vi "WildBugChilGru.vi"() -> ()   [LabVIEW 2014]
uses:
  <vilib>/Utility/miscctls.llb/LVPointTypeDef.ctl
  <vilib>/Utility/xml.llb/Write to XML File(string).vi
  <vilib>/Platform/browser.llb/Open URL in Default Browser (string).vi
  <vilib>/Instr/_visa.llb/VISA Configure Serial Port (Instr).vi
  <vilib>/Analysis/3filter.llb/IIR Filter (DBL).vi
  <vilib>/gmath/NI_Gmath.lvlib
  <vilib>/Analysis/NI_AALBase.lvlib
panel:
  in  "Fahrzeugdaten":string
  out "Ergebnis":string
  out "Pmax":string="0,0 PS"
  in  "Drucken":bool
  in  "Speichern":bool
  in  "Start":bool
  in  "Ende":bool
  in  "Spenden":bool
  in  "Registerkarte":T1(tab)
  in  "Zündung [Imp/U]":dbl=1.0
  in  "Übersetzung ermitteln aus":T2(ring)
  in  "Getriebe [1:]":dbl=4.0
  in  "Reifenumfang [m]":dbl=1.2
  in  "Dauer [s]":dbl=5.0
  in  "nKuWe/nRolle":dbl=1.0 format="%#.3f"
  in  "Lufttemperatur [°C]":dbl format="%#.1g"
  in  "Luftdruck [mbar]":dbl=1013.45
  in  "Messung Klimadaten":bool=TRUE
  in  "v vom Gas [km/h]":dbl=5000.0
  in  "Gleitender Mittelwert":u8=35
  in  "Differenzenquotient":u8=12
  in  "n vom Gas [1/min]":dbl=5000.0
  in  "Rollengeber [Inkr/U]":u16=200
  in  "Rollenumfang [m]":dbl=0.613
  in  "Rollenträgheit [kgm²]":dbl=0.402
  in  "Recalc":bool
  in  "Leistung":bool=TRUE caption="Messung Klimadaten"
  out "Datenspeicher":T3={"Fahrzeugdaten"="", "date/time string"="", "Rolle [Inkr/U]"=200, "Rollenumfang [m]"=0.613, "Rollenträgheit [kgm²]"=0.402, "Zündung [Imp/U]"=1.0, "Getriebe [1:]"=4.0, "Reifenumfang [m] "=1.2, "element"=0.0, "Gl. Mittelwert"=35, "Differenzenquotient"=12, 0, "dT [s]"=0.0, "element"=0.0, "Lufttemperatur [°C]"=0.0, "Luftfeuchtigkeit [%]"=43.8, "Luftdruck [mbar]"=1013.45, "nRolle"=[], "nWelle"=[], "ArrayReserve1"=[], "ArrayReserve2"=[], "Übersetzung ermitteln aus"=0, "[s]"=5.0, "nmin [1/min]"=0.0, "nmax [1/min]"=0.0, "n vom Gas [1/min]"=5000.0, "dT-Array [s]"=[], [], "Boolesch"=TRUE, "Serielle Schnittstelle"="COM6", "nKuWe/nRolle"=1.0, "v vom Gas [km/h]"=5000.0}
  out "COM-Fehlerrate":string="0 / 0,0%"
  in  "Konfiguration:":bool
  out "Füllstand Lesepuffer":u64(slide)=1 scale=1.0..100.0
  out "Lesepuffer":string="\n"
  in  "Serielle Schnittstelle":refnum<visa-resource-name>="COM6"
  in  "Registerkarte 2":enum32{"Seite 1", "Seite 2"}(tab)
  out "Text Zündung":string
  out "Text Rolle":string
  in  "Reset Skalierung":bool
  out "Welle\n[1/min]":cluster{dbl, dbl}(knob) scale=0.0..14000.0
  out "Untersetzung\nermittelt":bool
  out "Hinterrad\n[km/h]":dbl(knob) scale=0.0..200.0
  out "XY-Graph":cluster{dbl[], dbl[]}[](graph)
  out "Untersetzung":dbl format="%#.3f"
  out "Untersetzung-Graph":dbl(graph)=198.99999999999997 caption="Untersetzung"
  # "Leistungsmessung:\n1. Drehzahl konstant halten\n2. START [F1]\n3. Drehzahl weiter halten\n4. bei GO: Vollgas\n5. vom Gas gehen"
  # "Untersetzung aus:"
  # "Eingabe <> Messen"
  # "Tacho <> Leistung"
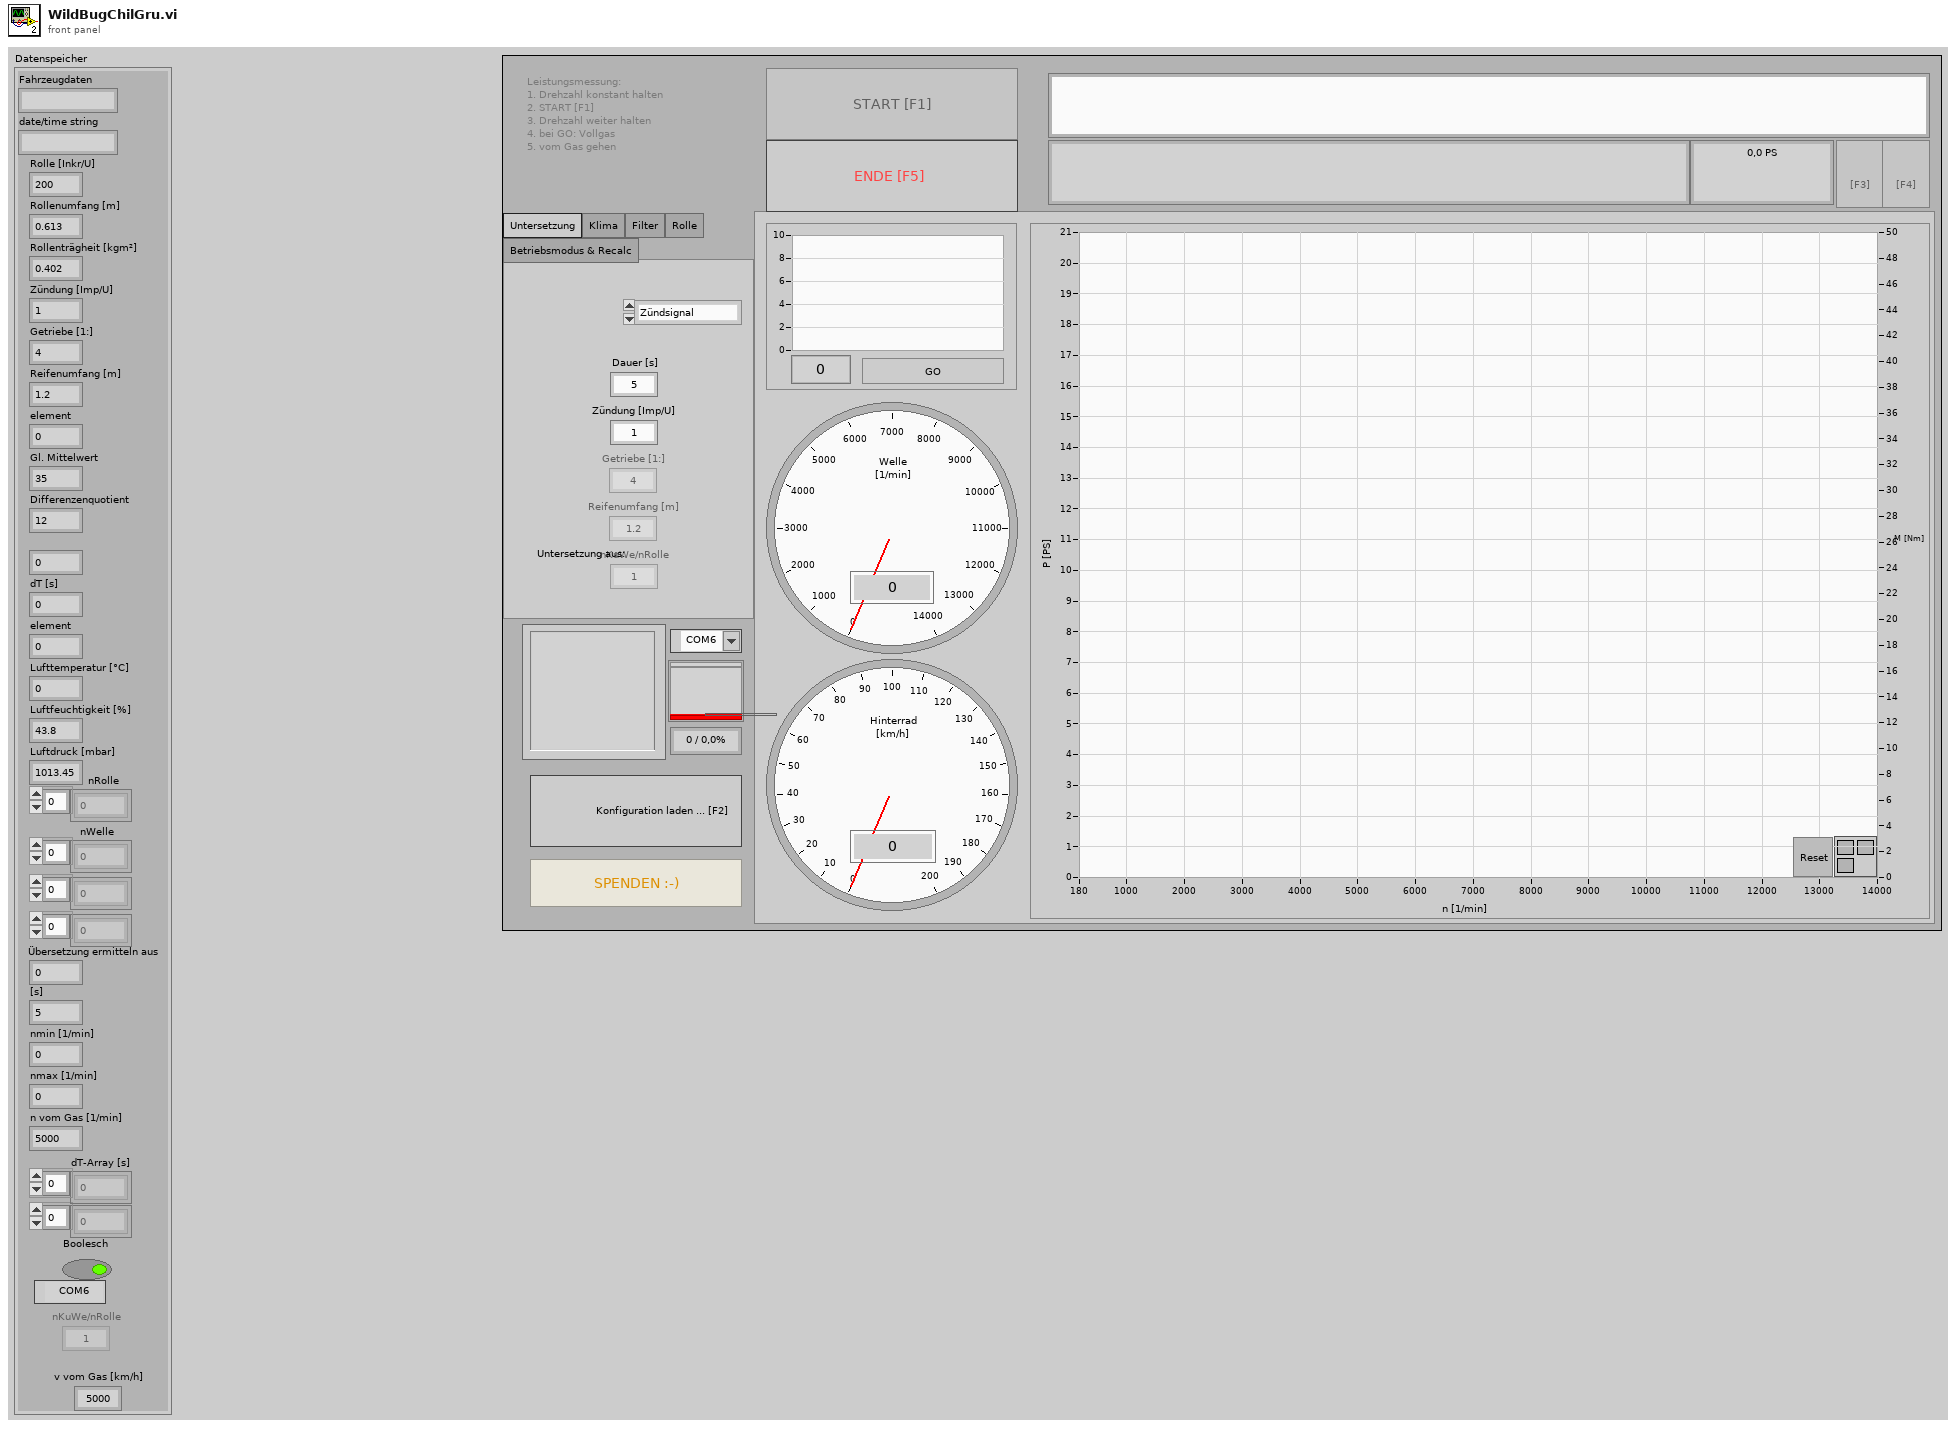
[diagram p1: front panel]
types:
  T1 = enum32{"Untersetzung", "Klima", "Filter", "Rolle", "Betriebsmodus & Recalc"}
  T2 = enum8{"Zündsignal", "Getriebe & Reifen", "nKuWe / nRolle", "Vario (km/h)"}
  T3 = cluster{"Fahrzeugdaten":string, "date/time string":string, "Rolle [Inkr/U]":u16, "Rollenumfang [m]":dbl, "Rollenträgheit [kgm²]":dbl, "Zündung [Imp/U]":dbl, "Getriebe [1:]":dbl, "Reifenumfang [m] ":dbl, "element":dbl, "Gl. Mittelwert":u8, "Differenzenquotient":u8, u8, "dT [s]":dbl, "element":dbl, "Lufttemperatur [°C]":dbl, "Luftfeuchtigkeit [%]":dbl, "Luftdruck [mbar]":dbl, "nRolle":dbl[], "nWelle":dbl[], "ArrayReserve1":dbl[], "ArrayReserve2":dbl[], "Übersetzung ermitteln aus":u8, "[s]":dbl, "nmin [1/min]":dbl, "nmax [1/min]":dbl, "n vom Gas [1/min]":dbl, "dT-Array [s]":dbl[], i32[], "Boolesch":bool, "Serielle Schnittstelle":refnum<visa-resource-name>, "nKuWe/nRolle":dbl, "v vom Gas [km/h]":dbl}
  T4 = enum8{"Enabled", "Disabled", "Disabled and Grayed Out"}
  T5 = cluster{"Fahrzeugdaten":string, "date/time string":string, "Rollengeber [Inkr/U]":u16, "Rollenumfang [m]":dbl, "Rollenträgheit [kgm²]":dbl, "Zündung [Imp/U]":dbl, "Getriebe [1:]":dbl, "Reifenumfang [m] ":dbl, "mean value":dbl, "Gleitender Mittelwert":u8, "Differenzenquotient":u8, u8, dbl, "Numerisch":dbl, "Lufttemperatur [°C]":dbl, dbl, "Luftdruck [mbar]":dbl, dbl[], dbl[], dbl[], dbl[], "Übersetzung ermitteln aus":enum8{"Zündsignal", "Getriebe & Reifen", "nKuWe / nRolle", "Vario (km/h)"}, "Dauer [s]":dbl, dbl, dbl, "n vom Gas [1/min]":dbl, dbl[], i32[], "Messung Klimadaten":bool, "VISA-Referenz (Ausgang)":refnum<visa-resource-name>, "nKuWe/nRolle":dbl, "v vom Gas [km/h]":dbl}
  T6 = typedef "LVPointTypeDef.ctl" = cluster{"Horizontal":i16, "Vertical":i16}
  T7 = enum32{"invalid app kind", "Development System", "Run Time System", "Student Edition", "Embedded LabVIEW", "Evaluation", "Custom"}
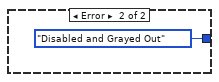
[diagram p8: hidden frame]
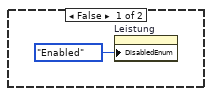
[diagram p9: hidden frame]
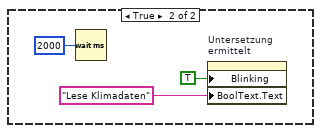
[diagram p10: hidden frame]
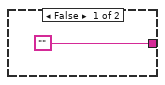
[diagram p12: hidden frame]
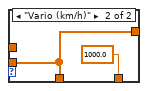
[diagram p15: hidden frame]
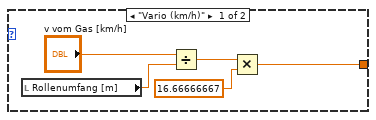
[diagram p16: hidden frame]
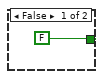
[diagram p17: hidden frame]
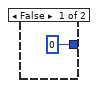
[diagram p19: hidden frame]
diagram:
  n1 = while {
    stop <- w5 stop-if-true
    n2 = local read "Leistung"() -> (w3:bool)
    n3 = Wait (ms)(milliseconds to wait=u32 10) -> ()  [unwired: 1 out]
    n4 = case shown="False" w3 {
      frame False {
        n5 = control-ref of="Welle\n[1/min]"() -> (w9:refnum<vi>)
        n6 = control-ref of="Hinterrad\n[km/h]"() -> (w8:refnum<vi>)
        n7 = control-ref of="Ende"() -> (w7:refnum<vi>)
        n8 = control-ref of="Leistung"() -> (w6:refnum<vi>)
        n9 = call "Tachomodus (SubVI).vi"("Leistung"=w6, "Stopp"=w7, "Hinterrad"=w8, "Welle"=w9) -> ()  [unwired: 8 in]
      }
      frame True {
      }
    }
    n10 = local read "Ende"() -> (w5:bool)
  }
  n11 = while {
    stop <- w13 stop-if-true
    n12 = local read "Start"() -> (w14:bool)
    n13 = Not(x="Leistung") -> (.not. x?=w10:bool)
    n14 = case shown="True" w14 {
      tunnel: "Leistung" -> [_ w23]
      frame False {
        n15 = property on="Leistung" class="Bool. (strikt)"("DisabledEnum"=T4."Enabled" ("Deaktiviert")) -> ()  [unwired: 2 in, 2 out]
      }
      frame True {
        n16 = flat-sequence {
          tunnel: [w115] -> w101
          tunnel: [w114] -> w100
          tunnel: [w112] -> w99
          tunnel: w23 -> [w110]
          tunnel: w101 -> [w129]
          tunnel: w100 -> [w133]
          tunnel: [0] -> w98
          tunnel: [1.0 ("element")] -> w97
          tunnel: [w131] -> w96
          tunnel: [w142] -> w95
          tunnel: [0] -> w94
          tunnel: [w131] -> w93
          tunnel: [-5] -> w92
          tunnel: [w139] -> w91
          tunnel: [w137] -> w90
          tunnel: [w136] -> w89
          tunnel: [0.0] -> w88
          tunnel: [w129] -> w87
          tunnel: [w133] -> w86
          tunnel: w99 -> [w132]
          tunnel: [w132] -> w85
          tunnel: [w170] -> w84
          tunnel: [w169] -> w83
          tunnel: [w168] -> w82
          tunnel: [w167] -> w81
          tunnel: [w166] -> w80
          tunnel: [w165] -> w79
          tunnel: [w164] -> w78
          tunnel: [w163] -> w77
          tunnel: [w162] -> w76
          tunnel: [w161] -> w75
          tunnel: [w160] -> w74
          tunnel: [w159] -> w22
          tunnel: [w158] -> w21
          tunnel: w98 -> [w170]
          tunnel: w97 -> [w169]
          tunnel: w96 -> [w168]
          tunnel: w95 -> [w167]
          tunnel: w94 -> [w166]
          tunnel: w93 -> [w165]
          tunnel: w92 -> [w164]
          tunnel: w91 -> [w163]
          tunnel: w90 -> [w162]
          tunnel: w89 -> [w161]
          tunnel: w88 -> [w160]
          tunnel: w87 -> [w156]
          tunnel: w86 -> [w155]
          tunnel: w85 -> [w157]
          tunnel: w84 -> [w187]
          tunnel: w83 -> [w186]
          tunnel: w82 -> [w185]
          tunnel: w81 -> [w184]
          tunnel: w80 -> [w183]
          tunnel: w79 -> [w182]
          tunnel: w78 -> [w181]
          tunnel: w77 -> [w180]
          tunnel: w76 -> [w179]
          tunnel: w75 -> [w178]
          tunnel: w74 -> [w177]
          tunnel: [w187] -> w73
          tunnel: [w186] -> w72
          tunnel: [w185] -> w71
          tunnel: [w184] -> w70
          tunnel: [w183] -> w69
          tunnel: [w182] -> w68
          tunnel: [w181] -> w67
          tunnel: [w180] -> w66
          tunnel: [w179] -> w65
          tunnel: [w178] -> w64
          tunnel: [w177] -> w63
          tunnel: [w176] -> w62
          tunnel: [w175] -> w61
          tunnel: [w173] -> w60
          tunnel: w22 -> [w176]
          tunnel: w21 -> [w175]
          tunnel: ["Gleitender Mittelwert"] -> w32
          tunnel: [w193] -> w33
          tunnel: [w192] -> w34
          tunnel: [w212] -> w35
          tunnel: [w206] -> w30
          tunnel: [w205] -> w31
          tunnel: [w213] -> w36
          tunnel: [w214] -> w37
          tunnel: [w215] -> w39
          tunnel: [w216] -> _
          tunnel: [w217] -> w41
          tunnel: [w218] -> w42
          tunnel: [w219] -> w55
          tunnel: [w220] -> w18
          tunnel: [w221] -> w57
          tunnel: [w222] -> w58
          tunnel: [w223] -> w59
          tunnel: w73 -> [w223]
          tunnel: w72 -> [w222]
          tunnel: w71 -> [w221]
          tunnel: w70 -> [w220]
          tunnel: w69 -> [w219]
          tunnel: w68 -> [w218]
          tunnel: w67 -> [w217]
          tunnel: w66 -> [w216]
          tunnel: w65 -> [w215]
          tunnel: w64 -> [w214]
          tunnel: w63 -> [w213]
          tunnel: w62 -> [w208]
          tunnel: w61 -> [w207]
          tunnel: w60 -> [w212]
          tunnel: [w199] -> w20
          tunnel: [w200] -> w19
          frame #0 {
            w120 = u16 0 items=["None", "XON/XOFF", "RTS/CTS", "XON/XOFF & RTS/CTS", "DTR/DSR", "XON/XOFF & DTR/DSR"] ("flow control (0:none)")
            w121 = u16 10 items=["1.0"=10, "1.5"=15, "2.0"=20] ("stop bits (10: 1 bit)")
            w113 = FALSE  # Enable Termination Char (T)
            w116 = u32 10000  # timeout (10sec)
            n17 = And(x="Messung Klimadaten", y=w110) -> (x .and. y?=w112:bool)
            n18 = call-poly "VISA Configure Serial Port"("VISA resource name"="Serielle Schnittstelle", "timeout (10sec)"=w116, "Enable Termination\nChar (T)"=w113, "baud rate (9600)"=u32 115200 ("baudrate (250000)"), "data bits (8)"=u16 8, "parity (0:none)"=enum16{"None", "Odd", "Even", "Mark", "Space"}."None", "stop bits (10: 1 bit)"=w121, "flow control (0:none)"=w120) -> ("VISA resource name out"=w118:refnum<visa-resource-name>, "error out"=w117:errorcluster)  [unwired: 6 in]
            n19 = VISA Clear(VISA resource name=w118, error in (no error)=w117) -> (VISA resource name out=w115:refnum<visa-resource-name>, error out=w114:errorcluster)
          }
          frame #1 {
            w130 = T4."Disabled and Grayed Out" ("Deaktiviert")
            w135 = 0.0  # Graphen löschen
            w138 = 0
            w143 = 0.0
            w131 = FALSE
            w136 = ""
            n20 = case shown="False" w132 {
              frame False {
                n21 = property on="Untersetzung\nermittelt" class="Bool. (strikt)"("Blinking"=TRUE ("Blinkend"), "BoolText.Text"="Initialisiere" ("Beschriftung.Text")) -> ()  [unwired: 2 in, 2 out]
              }
              frame True {
                n22 = Wait (ms)(milliseconds to wait=u32 2000 ("Zu wartende ms")) -> ()  [unwired: 1 out]
                n23 = property on="Untersetzung\nermittelt" class="Bool. (strikt)"("Blinking"=TRUE ("Blinkend"), "BoolText.Text"="Lese Klimadaten" ("Beschriftung.Text")) -> ()  [unwired: 2 in, 2 out]
              }
            }
            n24 = Build Array(w135) -> (w125:dbl[])
            n25 = property on="Untersetzung-Graph" class="SVDiagr (strikt)"("History Data"=w125) -> ()  [unwired: 2 in, 2 out]
            n26 = property on="Drucken" class="Bool. (strikt)"("DisabledEnum"=w130) -> ()  [unwired: 2 in, 2 out]
            n27 = property on="Übersetzung ermitteln aus" class="Enum (strikt)"("DisabledEnum"=w130) -> ()  [unwired: 2 in, 2 out]
            n28 = property on="Konfiguration:" class="Bool. (strikt)"("DisabledEnum"=w130) -> ()  [unwired: 2 in, 2 out]
            n29 = property on="Ende" class="Bool. (strikt)"("DisabledEnum"=w130) -> ()  [unwired: 2 in, 2 out]
            n30 = property on="Leistung" class="Bool. (strikt)"("DisabledEnum"=w130) -> ()  [unwired: 2 in, 2 out]
            n31 = property on="Speichern" class="Bool. (strikt)"("DisabledEnum"=w130) -> ()  [unwired: 2 in, 2 out]
            n32 = local write "Pmax"(w136) -> ()
            n33 = local write "COM-Fehlerrate"(w136) -> ()
            n34 = local write "Ergebnis"(w136) -> ()
            n35 = Bundle(w125, w125) -> (w127:cluster{dbl[], dbl[]})  [unwired: 1 in]
            n36 = Bundle(w125, w125) -> (w126:cluster{dbl[], dbl[]})  [unwired: 1 in]
            n37 = Build Array(w127, w126) -> (w128:cluster{dbl[], dbl[]}[])
            n38 = local write "XY-Graph"(w128) -> ()
            n39 = Initialize Array(w138, w138) -> (w137:i32[])
            n40 = Initialize Array(0.0 ("y"), 0) -> (w139:dbl[])
            n41 = Initialize Array(w143, w143) -> (w142:dbl[])
          }
          frame #2 {
            n42 = control-ref of="Lufttemperatur [°C]"() -> (w153:refnum<vi>)
            n43 = control-ref of="Luftdruck [mbar]"() -> (w154:refnum<vi>)
            n44 = call "MessungKlimadaten(SubVI).vi"("Boolesch"=w157, "Fehler (Eingang, kein Fehler)"=w155, "VISA resource name out"=w156, "Lufttemperatur [°C] (Eingang)"=w153, "Luftdruck [mbar] (Eingang)"=w154) -> ("Fehler (Ausgang)"=w158:errorcluster, "VISA-Referenz (Ausgang)"=w159:refnum<visa-resource-name>)  [unwired: 5 in]
          }
          frame #3 {
            n45 = Wait (ms)(milliseconds to wait=u32 2000 ("Zu wartende ms")) -> ()  [unwired: 1 out]
            n46 = call "KorrekturfaktorDin70020 (SubVI).vi"("Lufttemperatur [°C]"="Lufttemperatur [°C]", "Luftdruck [mbar]"="Luftdruck [mbar]") -> ("Numerisch"=w173:dbl)  [unwired: 9 in]
          }
          frame #4 {
            w188 = 0
            n47 = Concatenate Strings("m" ("String"), "\n") -> (w211:string)
            n48 = property on="Untersetzung\nermittelt" class="Bool. (strikt)"("Blinking"=FALSE ("Blinkend")) -> ()  [unwired: 2 in, 2 out]
            n49 = VISA Write(VISA resource name=w208, write buffer=w211, error in (no error)=w207) -> (VISA resource name out=w205:refnum<visa-resource-name>, error out=w206:errorcluster)  [unwired: 1 out]
            n50 = property on="XY-Graph" class="XYGraph (strikt)"("ActYScl"=w188, "YScale.ScaleFit"=w188, "ActYScl"=1, "YScale.ScaleFit"=w188, "XScale.ScaleFit"=w188, "Smooth Update"=TRUE ("Kontinuierliche Aktualisierung")) -> ()  [unwired: 2 in, 2 out]
            n51 = local read "Differenzenquotient"() -> (w203:u8)
            n52 = Divide(x="Gleitender Mittelwert", y=2) -> (x/y=w197:dbl)
            n53 = Round Toward -Infinity(1:w197) -> (0:w198:dbl)
            n54 = call <vilib>:"Smoothing Filter Coefficients.vi"("shape"=1, "half-width"=w198, "type"=0) -> ("forward coefficients"=w193:dbl[], "reverse coefficients"=w192:dbl[])  [unwired: 6 in, 1 out]
            n55 = call <vilib>:"Smoothing Filter Coefficients.vi"("shape"=0, "half-width"=w203, "type"=0) -> ("forward coefficients"=w200:dbl[], "reverse coefficients"=w199:dbl[])  [unwired: 6 in, 1 out]
          }
        }
        n56 = while {
          tunnel: w31 -> [w387]
          tunnel: w30 -> [w386]
          shift-right: [w444] -> _
          shift-left: w37 -> [w400]
          shift-right: [w439] -> _
          shift-left: w36 -> [w443]
          shift-right: [w438] -> _
          shift-left: w36 -> [w442]
          shift-right: [w404] -> _
          shift-left: w36 -> [w441]
          shift-right: [w424] -> _
          shift-left: w59 -> [w440]
          shift-right: [w359] -> w44
          shift-left: w58 -> [_]
          shift-right: [w409] -> w48
          shift-left: w36 -> [w381]
          shift-right: [w377] -> w46
          shift-left: w36 -> [w406]
          shift-right: [w405] -> _
          shift-left: w18 -> [w435]
          shift-right: [w380] -> _
          shift-left: w57 -> [w375]
          shift-right: [w388] -> _
          shift-left: w18 -> [_]
          shift-right: [w365] -> _
          shift-left: w18 -> [_]
          shift-right: [w432] -> w47
          shift-left: w18 -> [w430]
          shift-right: [w431] -> _
          shift-left: w18 -> [w366]
          shift-right: [w371] -> w54
          shift-left: w18 -> [w429]
          shift-right: [w423] -> _
          shift-left: w18 -> [w427]
          shift-right: [w422] -> w24
          shift-left: w18 -> [w428]
          shift-right: [w370] -> w53
          shift-left: w18 -> [w426]
          shift-right: [w369] -> w52
          shift-left: w18 -> [w425]
          tunnel: [w421] -> w56
          shift-right: [w417] -> w51
          shift-left: w55 -> [w419]
          tunnel: [w420] -> w27
          tunnel: [w374] -> w50
          tunnel: ["Rollenumfang [m]"] -> w49
          tunnel: ["Rollenumfang [m]"] -> w43
          shift-right: [w416] -> _
          shift-left: w42 -> [w385]
          shift-right: [w410] -> _
          shift-left: w41 -> [w415]
          shift-right: [w411] -> _
          shift-left: w36 -> [w414]
          shift-right: [w412] -> _
          shift-left: w36 -> [w413]
          shift-right: [w384] -> w40
          shift-left: w18 -> [w408]
          shift-right: [w403] -> _
          shift-left: _ -> [w402]
          shift-right: [w407] -> w38
          shift-left: w39 -> [w401]
          tunnel: [w399] -> w28
          tunnel: w35 -> [w359]
          tunnel: w34 -> [w388]
          tunnel: w33 -> [w365]
          tunnel: w32 -> [w392]
          tunnel: w20 -> [w383]
          tunnel: w19 -> [w382]
          tunnel: [u8 0 ("X-Achse.Achsenanpassung")] -> _
          shift-right: [w357] -> w16
          shift-left: w18 -> [w360]
          i -> [w362]
          stop <- w421 stop-if-true
          n57 = property class="Instr"(reference=w387, error in=w386) -> (reference out=w395:refnum<visa-resource-name>, error out=w394:errorcluster, "Serial Settings:Number of Bytes at Serial Port"=w397:u32)
          n58 = Greater?(x=w397, y=u32 1 ("min. Bytes")) -> (0:w393:bool)
          n59 = case shown="True" w393 {
            tunnel: w397 -> [_ w479]
            tunnel: [u32 0 ("Bytes at Port") w479] -> w396
            frame False {
            }
            frame True {
            }
          }
          n60 = control-ref of="Füllstand Lesepuffer"() -> (w373:refnum<vi>)
          n61 = call "Stringhandling(SubVI)0.0.2.vi"("Slide (Eingang)"=w373, "Numerisch (Eingang)"=w440, "VISA-Referenz (Eingang)"=w395, "MessFrequenz [Hz]"=w441, "Bytes at Port"=w396, "Fehler (Eingang, kein Fehler)"=w394, "Cyclecounter (Eingang)"=w402, "Rolle[Hz]"=w442, "String (Eingang)"=w400, "Zündung [Hz] (Eingang)"=w443) -> ("Lesepuffer"=→"Lesepuffer":string, "Numerisch (Ausgang)"=w424:i32, "String (Ausgang)"=w444:string, "VISA-Referenz (Ausgang)"=w399:refnum<visa-resource-name>, "Zündung [Hz] (Ausgang)"=w439:dbl, "Rolle [Hz]"=w438:dbl, "Messfrequenz [Hz]"=w404:dbl, "Cyclecounter (Ausgang)"=w403:i32, "Fehler (Ausgang)"=w420:errorcluster)  [unwired: 1 in]
          "Füllstand Lesepuffer" <- w424
          n62 = Not Equal?(x=w402, y=w403) -> (x != y?=w389:bool)
          n63 = case shown="True" w389 {
            tunnel: w415 -> [w483 w494]
            tunnel: [w483 w506] -> w410
            tunnel: w414 -> [w482 w505]
            tunnel: [w482 w491] -> w411
            tunnel: w413 -> [w481 w504]
            tunnel: [w481 w492] -> w412
            tunnel: w403 -> [_ w490]
            tunnel: w401 -> [w480 w489]
            tunnel: [w480 w493] -> w407
            frame False {
            }
            frame True {
              n64 = Build Array (concatenate)(w489, w490) -> (w493:i32[])
              n65 = Greater Or Equal To 0?(x=w494) -> (x >= 0?=w495:bool)
              n66 = case shown="True" w495 {
                tunnel: [w507 w518] -> w491
                tunnel: [w507 w519] -> w492
                tunnel: [w508 w510] -> w506
                tunnel: w505 -> [_ w512]
                tunnel: w504 -> [_ w520]
                tunnel: w490 -> [w508 w509]
                tunnel: w494 -> [_ w510]
                frame False {
                  w507 = 1.0
                }
                frame True {
                  w516 = 65536.0
                  n67 = Add(x=w510, y=w512) -> (x+y=w511:dbl)
                  n68 = Divide(x=w511, y=w516) -> (x/y=w521:dbl)
                  n69 = Increment(x=w520) -> (x+1=w519:dbl)
                  n70 = Round Toward -Infinity(1:w521) -> (0:w517:dbl)
                  n71 = Multiply(x=w517, y=w516) -> (x*y=w515:dbl)
                  n72 = Add(x=w515, y=w509) -> (x+y=w514:dbl)
                  n73 = Increment(x=w514) -> (x+1=w513:dbl)
                  n74 = Subtract(x=w513, y=w510) -> (x-y=w518:dbl)
                }
              }
              n75 = Subtract(x=w491, y=w492) -> (x-y=w486:dbl)
              n76 = Decrement(x=w486) -> (x-1=w485:dbl)
              n77 = Max & Min(x=0, y=w485) -> (max(x,y)=w484:dbl)  [unwired: 1 out]
              n78 = Divide(x=w484, y=w491) -> (x/y=w498:dbl)
              n79 = Greater Than 0?(x=w484) -> (x > 0?=w488:bool)
              n80 = Select(t=u32 16711680, s=w488, f=u32 0) -> (s? t:f=w499:u32)
              n81 = Multiply(x=w498, y=100.0) -> (x*y=w496:dbl)
              n82 = property on="COM-Fehlerrate" class="Str"("Text.TextColor"=w499) -> ()  [unwired: 2 in, 2 out]
              n83 = Format Into String(format string="%d / %.1f%%" ("Format-String"), w484, w496) -> (resulting string=→"COM-Fehlerrate":string)  [unwired: 2 in, 1 out]
            }
          }
          n84 = local read "Übersetzung ermitteln aus"() -> (w356:T2)
          n85 = case "Case-Struktur" shown="True" w389 {
            tunnel: w439 -> [w701 w717]
            tunnel: w438 -> [w700 w716]
            tunnel: [w701 w702] -> w437
            tunnel: [w700 w715] -> w436
            tunnel: w404 -> [_ w710]
            tunnel: w381 -> [w699 _]
            tunnel: [w699 w709] -> w409
            tunnel: w406 -> [_ w714]
            tunnel: "Rollenumfang [m]" -> [_ w713]
            tunnel: w356 -> [_ w706]
            frame False {
            }
            frame True {
              w722 = 60.0 ("y")
              n86 = Reciprocal "Abtastzeit [s]"(x=w710) -> (1/x=w709:dbl)
              n87 = Divide "R [1/s]"(x=w716, y="Rollengeber [Inkr/U]") -> (x/y=w721:dbl)
              n88 = Divide(x=w717, y="Zündung [Imp/U]") -> (x/y=w720:dbl)
              n89 = Multiply "nZ gemessen [1/min]"(x=w720, y=w722) -> (x*y=w702:dbl)
              n90 = Multiply "nR [1/min]"(x=w722, y=w721) -> (x*y=w715:dbl)
              n91 = Multiply "nZ berechnet [1/min]"(x=w715, y=w714) -> (x*y=w704:dbl)
              n92 = Multiply "[m/min]"(x=w715, y=w713) -> (x*y=w718:dbl)
              n93 = case shown="Standard" w706 {
                tunnel: [w724 w725] -> w705
                tunnel: w704 -> [w724 w726]
                tunnel: [w723 w726] -> w703
                tunnel: w702 -> [w723 w725]
                frame Default {
                }
                frame "Vario (km/h)" {
                }
              }
              n94 = Multiply "[km/h]"(x=w718, y=0.06) -> (x*y=→"Hinterrad\n[km/h]":dbl)
              n95 = Bundle(w705, w703) -> (→"Welle\n[1/min]":cluster{dbl, dbl})  [unwired: 1 in]
            }
          }
          n96 = case shown="Standard" w356 {
            tunnel: [w470 "n vom Gas [1/min]"] -> w374
            frame "Vario (km/h)" {
              n97 = local read "Rollenumfang [m]"() -> (w471:dbl)
              n98 = Divide(x="v vom Gas [km/h]", y=w471) -> (x/y=w469:dbl)
              n99 = Multiply(x=w469, y=16.66666667) -> (x*y=w470:dbl)
            }
            frame Default {
            }
          }
          n100 = case shown="True" w389 {
            tunnel: w437 -> [_ w551]
            tunnel: w436 -> [_ w616]
            tunnel: "Rollenumfang [m]" -> [_ w619]
            tunnel: [w534 w592] -> w377
            tunnel: w406 -> [w523 w592]
            tunnel: w375 -> [w535 w554]
            tunnel: w435 -> [w536 w622]
            tunnel: [w535 w584] -> w380
            tunnel: [w536 w621] -> w405
            tunnel: w388 -> [_ w618]
            tunnel: w365 -> [_ w617]
            tunnel: [w533 w556] -> w432
            tunnel: [w532 w564] -> w431
            tunnel: w430 -> [w533 w615]
            tunnel: w366 -> [w532 _]
            tunnel: w392 -> [_ w573]
            tunnel: [w531 w597] -> w371
            tunnel: w429 -> [w531 _]
            tunnel: [w530 w563] -> w423
            tunnel: w427 -> [w530 _]
            tunnel: [w529 w598] -> w422
            tunnel: w428 -> [w529 _]
            tunnel: [w528 w609] -> w370
            tunnel: w426 -> [w528 _]
            tunnel: [w527 w608] -> w369
            tunnel: w425 -> [w527 _]
            tunnel: w359 -> [_ w601]
            tunnel: w419 -> [w526 w596]
            tunnel: w374 -> [_ w586]
            tunnel: [w526 w595] -> w417
            tunnel: w385 -> [w525 w591]
            tunnel: [w525 w590] -> w416
            tunnel: w409 -> [_ w589]
            tunnel: [w524 w557] -> w384
            tunnel: w408 -> [w524 w588]
            tunnel: w383 -> [_ w571]
            tunnel: w382 -> [_ w570]
            tunnel: w360 -> [w522 w553]
            tunnel: [w522 w552] -> w357
            frame False {
              n101 = case shown="False" w535 {
                tunnel: w536 -> [w543 _]
                tunnel: [w537 w550] -> w534
                tunnel: w523 -> [_ w550]
                frame False {
                  n102 = call <vilib>:"Measures of Mean.vi"("percent (trim)"=20.0, "type"=3, "x array"=w543) -> ("mean value"=w538:dbl)  [unwired: 7 in, 1 out]
                  n103 = local read "Übersetzung ermitteln aus"() -> (w540:T2)
                  n104 = Equal To 0? "aus Zündsignal?"(x=w540) -> (x = 0?=w539:bool)
                  n105 = case shown="True" w539 {
                    tunnel: w538 -> [w544 w549]
                    tunnel: [w544 w545] -> w537
                    frame False {
                    }
                    frame True {
                      w546 = 1000.0
                      n106 = Multiply(x=w549, y=w546) -> (x*y=w548:dbl)
                      n107 = Round To Nearest(number=w548) -> (nearest integer value=w547:dbl)
                      n108 = Divide(x=w547, y=w546) -> (x/y=w545:dbl)
                    }
                  }
                }
                frame True {
                }
              }
            }
            frame True {
              w604 = 0.00135962  # [W] in [PS]
              w611 = 0.10471975511965978  # 2*Pi/60
              n109 = Not(x=w554) -> (.not. x?=w560:bool)
              n110 = local read "Leistung"() -> (w559:bool)
              n111 = Or(x=w559, y=w560) -> (x .or. y?=w558:bool)
              n112 = Square(x=w592) -> (x^2=w610:dbl)
              n113 = local read "Übersetzung ermitteln aus"() -> (w561:T2)
              n114 = case shown="False" w558 {
                tunnel: w616 -> [_ w634]
                tunnel: w615 -> [w624 w633]
                tunnel: w589 -> [_ w632]
                tunnel: w588 -> [w625 w631]
                tunnel: [w624 w630] -> w556
                tunnel: [w625 w629] -> w557
                tunnel: w553 -> [w623 w628]
                tunnel: [w623 w627] -> w552
                tunnel: w551 -> [_ w626]
                frame False {
                }
                frame True {
                  n115 = Build Array (concatenate) "nRolle in Array einf."(w633, w634) -> (w630:dbl[])
                  n116 = Build Array (concatenate) "dT in Array einf."(w631, w632) -> (w629:dbl[])
                  n117 = Build Array (concatenate) "nWelle in Array einf."(w628, w626) -> (w627:dbl[])
                }
              }
              n118 = Divide(x="Rollenträgheit [kgm²]", y=w610) -> (x/y=w602:dbl)
              n119 = case shown="\"Zündsignal\"" w561 {
                tunnel: w551 -> [w691 _ _ _]
                tunnel: w616 -> [w690 _ _ _]
                tunnel: [w689 w695 "nKuWe/nRolle" 1.0] -> w620
                tunnel: w619 -> [_ w696 _ _]
                frame "Zündsignal" {
                  n120 = Divide(x=w691, y=w690) -> (x/y=w689:dbl)
                }
                frame "Getriebe & Reifen" {
                  n121 = Divide(x=w696, y="Reifenumfang [m]") -> (x/y=w694:dbl)
                  n122 = Multiply(x=w694, y="Getriebe [1:]") -> (x*y=w695:dbl)
                }
                frame "nKuWe / nRolle" {
                }
                frame "Vario (km/h)" {
                }
              }
              n123 = Multiply(x=w602, y=w601) -> (x*y=w600:dbl)
              n124 = local read "Differenzenquotient"() -> (w569:u8)
              n125 = Multiply(x=2, y=w569) -> (x*y=w567:i32)
              n126 = Increment(x=w567) -> (x+1=w565:i32)
              n127 = Index Array(array=w556, index=1 ("Index")) -> (element=w582:dbl)
              n128 = Index Array(array=w557, index=1 ("Index")) -> (element=w576:dbl)
              n129 = Initialize Array(w582, w573) -> (w581:dbl[])
              n130 = Initialize Array(w576, w565) -> (w574:dbl[])
              n131 = Insert Into Array(array=w556, index=0 ("Index"), new element=w581) -> (w579:dbl[])
              n132 = Insert Into Array(array=w557, index=0 ("Index"), new element=w574) -> (w572:dbl[])
              n133 = call-poly <vilib>:"IIR Filter.vi"("Forward Coefficients"=w617, "Reverse Coefficients"=w618, "X"=w579) -> ("Filtered X"=w578:dbl[])  [unwired: 1 in, 1 out]
              n134 = call-poly <vilib>:"IIR Filter.vi"("Forward Coefficients"=w570, "Reverse Coefficients"=w571, "X"=w572) -> ("Filtered X"=w566:dbl[])  [unwired: 1 in, 1 out]
              n135 = case shown="False" w554 {
                selector: w554 -> [_ w688]
                tunnel: w620 -> [w677 _]
                tunnel: w622 -> [w679 w687]
                tunnel: [w674 w688] -> w614
                tunnel: [w678 w687] -> w621
                tunnel: w591 -> [w676 w686]
                tunnel: [w674 w686] -> w590
                tunnel: w561 -> [w673 _]
                frame False {
                  n136 = Build Array (concatenate)(w679, w677) -> (w678:dbl[])
                  n137 = case shown="\"Zündsignal\"" w673 {
                    tunnel: ["Dauer [s]" 0.0 ("Dauer [s]")] -> w675
                    frame "Zündsignal" {
                      n138 = property on="Untersetzung\nermittelt" class="Bool. (strikt)"("Blinking"=TRUE ("Blinkend"), "BoolText.Text"="Ermittle Übersetzung" ("Boolescher Text.Text")) -> ()  [unwired: 2 in, 2 out]
                    }
                    frame Default {
                    }
                  }
                  n139 = call "Verstrichene Zeit"("Time Target (s)"=w675, "Reset"=w676) -> ("Time has Elapsed"=w674:bool)  [unwired: 10 in, 7 out]
                  n140 = case shown="True" w674 {
                    frame False {
                    }
                    frame True {
                      n141 = property on="Untersetzung\nermittelt" class="Bool. (strikt)"("Blinking"=FALSE ("Blinkend"), "BoolText.Text"="Go" ("Boolescher Text.Text")) -> ()  [unwired: 2 in, 2 out]
                    }
                  }
                  "Untersetzung-Graph" <- w677
                }
                frame True {
                }
              }
              n142 = Array Subset "Rolle gefiltert [1/min]"(array=w578, index=w573) -> (w564:dbl[])  [unwired: 1 in]
              n143 = Array Subset "dT gefiltert [s]"(array=w566, index=w565) -> (w562:dbl[])  [unwired: 1 in]
              n144 = Array Size "Array-Größe"(array=w564) -> (size(s)=w612:i32)
              n145 = Greater?(x=w612, y=w573) -> (0:w613:bool)
              n146 = Multiply(x=w564, y=w592) -> (x*y=w597:dbl[])
              n147 = Multiply(x=w597, y=w611) -> (x*y=w563:dbl[])
              n148 = And(x=w614, y=w613) -> (x .and. y?=w584:bool)
              n149 = Array Size "Array-Größe"(array=w563) -> (size(s)=w555:i32)
              n150 = Decrement(x=w555) -> (x-1=w599:i32)
              n151 = Select(t=w586, s=w584, f=1000000.0) -> (s? t:f=w587:dbl)
              n152 = Initialize Array(0.0 ("y"), 0) -> (w605:dbl[])
              n153 = for {
                N: w555 -> [_]
                tunnel: "Differenzenquotient" -> [w649]
                tunnel: w563 -> [w657]
                tunnel: w599 -> [w648]
                shift-right: [w654] -> w598
                shift-left: w605 -> [w655]
                tunnel: w597 -> [w652] mode=indexing
                tunnel: w596 -> [w641]
                tunnel: w587 -> [w651]
                tunnel: [w642] -> w595
                tunnel: w554 -> [w640]
                tunnel: w562 -> [w637] mode=indexing
                i -> [w638]
                stop <- w635 stop-if-true
                n154 = Subtract(x=w648, y=w649) -> (x-y=w650:i32)
                n155 = Multiply(x=w637, y=2.0) -> (x*y=w639:dbl)
                n156 = Subtract(x=w638, y=w649) -> (x-y=w670:i32)
                n157 = Add(x=w638, y=w649) -> (x+y=w664:i32)
                n158 = Greater Or Equal?(x=w638, y=w649) -> (x >= y?=w645:bool)
                n159 = Less Or Equal?(x=w638, y=w650) -> (x <= y?=w646:bool)
                n160 = Greater?(x=w652, y=w651) -> (0:w653:bool)
                n161 = Max & Min(x=w648, y=w664) -> (min(x,y)=w665:i32)  [unwired: 1 out]
                n162 = Max & Min(x=w670, y=0) -> (max(x,y)=w668:i32)  [unwired: 1 out]
                n163 = Subtract(x=w665, y=w638) -> (x-y=w666:i32)
                n164 = Subtract(x=w638, y=w668) -> (x-y=w667:i32)
                n165 = Max & Min(x=w667, y=w666) -> (min(x,y)=w658:i32)  [unwired: 1 out]
                n166 = Add(x=w638, y=w658) -> (x+y=w663:i32)
                n167 = Subtract(x=w638, y=w658) -> (x-y=w662:i32)
                n168 = Multiply(x=w658, y=w639) -> (x*y=w656:dbl)
                n169 = Index Array(array=w657, index=w663) -> (element=w660:dbl)
                n170 = Index Array(array=w657, index=w662) -> (element=w661:dbl)
                n171 = Subtract(x=w660, y=w661) -> (x-y=w659:dbl)
                n172 = Divide(x=w659, y=w656) -> (x/y=w647:dbl)
                n173 = Less Than 0?(x=w647) -> (x < 0?=w644:bool)
                n174 = Less Or Equal To 0?(x=w641) -> (x <= 0?=w643:bool)
                n175 = Build Array (concatenate)(w655, w647) -> (w654:dbl[])
                n176 = Compound Arithmetic op=AND(w644, w653, w643, w645, w646, w640) -> (w635:bool)
                n177 = case shown="False" w635 {
                  tunnel: w638 -> [_ w672]
                  tunnel: [w671 w672] -> w642
                  tunnel: w641 -> [w671 _]
                  frame False {
                  }
                  frame True {
                  }
                }
              }
              n178 = Multiply(x=w598, y=w600) -> (x*y=w609:dbl[])
              n179 = Multiply(x=w563, y=w609) -> (x*y=w603:dbl[])
              n180 = Multiply(x=w604, y=w603) -> (x*y=w608:dbl[])
            }
          }
          "Untersetzung\nermittelt" <- w380
          n181 = local read "Übersetzung ermitteln aus"() -> (w358:T2)
          n182 = Quotient & Remainder(x=w362, y=500) -> (x-y*floor(x/y)=w364:i32)  [unwired: 1 out]
          n183 = Equal To 0? "aus Zündsignal?"(x=w358) -> (x = 0?=w379:bool)
          n184 = Equal To 0?(x=w364) -> (x = 0?=w363:bool)
          n185 = local read "Leistung"() -> (w376:bool)
          n186 = And(x=w380, y=w379) -> (x .and. y?=w378:bool)
          n187 = case shown="True" w376 {
            tunnel: [FALSE w476] -> w418
            tunnel: w417 -> [_ w475]
            frame False {
            }
            frame True {
              n188 = Greater Than 0?(x=w475) -> (x > 0?=w476:bool)
            }
          }
          n189 = case shown="True" w363 {
            tunnel: w371 -> [_ w460]
            tunnel: w370 -> [_ w450]
            tunnel: w369 -> [_ w456]
            tunnel: w358 -> [_ w452]
            tunnel: "Rollenumfang [m]" -> [_ w459]
            tunnel: w357 -> [_ w449]
            frame False {
            }
            frame True {
              # "Skal-Y2"
              # "Skal-Y1"
              # "Skal-X"
              n190 = call "n2v (SubVI).vi"("Übersetzung ermitteln aus"=w452, "Array (Eingang)"=w460, "Rollenumfang [m]"=w459) -> ("Array (Ausgang)"=w453:dbl[])  [unwired: 7 in, 1 out]
              n191 = control-ref of="XY-Graph"() -> (w447:refnum<vi>)
              n192 = case shown="Standard" w452 {
                tunnel: [w465 w467] -> w451
                tunnel: w450 -> [w465 _]
                tunnel: w449 -> [_ w467]
                tunnel: [w465 w467] -> w448
                tunnel: [10.0 1000.0] -> w445
                frame Default {
                }
                frame "Vario (km/h)" {
                }
              }
              n193 = call "Scale_Graph_Y (SubVI).vi"("AktYSkl"=1, "Divisor"=w445, "Array"=w448, "Faktor"=1.8, "XYGraph (Eingang)"=w447) -> ()  [unwired: 7 in]
              n194 = call "Scale_Graph_Y (SubVI).vi"("AktYSkl"=0, "Divisor"=10.0, "Array"=w456, "Faktor"=1.0, "XYGraph (Eingang)"=w447) -> ()  [unwired: 7 in]
              n195 = Bundle("Array (Ausgang)"=w453, w451) -> (w461:cluster{"Array (Ausgang)":dbl[], dbl[]})  [unwired: 1 in]
              n196 = Bundle("Array (Ausgang)"=w453, w456) -> (w462:cluster{"Array (Ausgang)":dbl[], dbl[]})  [unwired: 1 in]
              n197 = call "Scale_Graph_X (SubVI).vi"("Array"=w453, "Übersetzung ermitteln aus"=w452, "XYGraph (Eingang)"=w447) -> ()  [unwired: 9 in]
              n198 = Build Array(w462, w461) -> (w463:cluster{"Array (Ausgang)":dbl[], dbl[]}[])
              n199 = local write "XY-Graph"(w463) -> ()
            }
          }
          n200 = Select(t=w377, s=w380, f=0.0) -> (s? t:f=→"Untersetzung":dbl)
          n201 = case shown="True" w378 {
            tunnel: w377 -> [_ w477]
            frame False {
            }
            frame True {
              n202 = local write "nKuWe/nRolle"(w477) -> ()
            }
          }
          n203 = local read "Start"() -> (w391:bool)
          n204 = Not(x=w391) -> (.not. x?=w390:bool)
          n205 = Or(x=w418, y=w390) -> (x .or. y?=w421:bool)
        }
        n206 = VISA Clear(VISA resource name=w28, error in (no error)=w27) -> (VISA resource name out=w25:refnum<visa-resource-name>, error out=w29:errorcluster)
        n207 = VISA Close(VISA resource name=w25, error in (no error)=w29) -> ()  [unwired: 1 out]
        n208 = case shown="True" w56 {
          tunnel: w54 -> [_ w333]
          tunnel: w53 -> [_ w338]
          tunnel: w52 -> [_ w337]
          tunnel: w51 -> [_ w321]
          tunnel: w24 -> [_ w334]
          tunnel: w50 -> [_ w332]
          tunnel: w49 -> [_ w295]
          tunnel: w44 -> [_ w308]
          tunnel: ["" w305] -> w45
          tunnel: w46 -> [_ w302]
          tunnel: w16 -> [_ w281]
          tunnel: w16 -> [_ w276]
          frame False {
          }
          frame True {
            w293 = 1
            w286 = 0
            w296 = 0.06
            n209 = Array Subset "P"(array=w337, length=w321) -> (w329:dbl[])  [unwired: 1 in]
            n210 = Array Subset "M"(array=w338, length=w321) -> (w330:dbl[])  [unwired: 1 in]
            n211 = Array Subset "alpha"(array=w334, length=w321) -> (w335:dbl[])  [unwired: 1 in]
            n212 = Array Subset "n"(array=w333, length=w321) -> (w331:dbl[])  [unwired: 1 in]
            n213 = property on="Ergebnis" class="Str"("Text.FontSize"=18) -> ()  [unwired: 2 in, 2 out]
            n214 = Array Size(array=w335) -> (size(s)=w336:i32)
            n215 = Array Max & Min "nWellemax [1/min]"(array=w276) -> (max value=w277:dbl)  [unwired: 3 out]
            n216 = for {
              N: w336 -> [w355]
              tunnel: w334 -> [w352]
              tunnel: w333 -> [w349]
              tunnel: w332 -> [w346]
              tunnel: [w344] -> w320
              i -> [w350]
              stop <- w345 stop-if-true
              n217 = Decrement(x=w355) -> (x-1=w354:i32)
              n218 = Subtract(x=w354, y=w350) -> (x-y=w344:i32)
              n219 = Index Array(array=w349, index=w344) -> (element=w348:dbl)
              n220 = Index Array(array=w352, index=w344) -> (element=w353:dbl)
              n221 = Less?(x=w348, y=w346) -> (x < y?=w347:bool)
              n222 = Less Or Equal To 0?(x=w353) -> (x <= 0?=w351:bool)
              n223 = And(x=w351, y=w347) -> (x .and. y?=w345:bool)
            }
            n224 = local read "Übersetzung ermitteln aus"() -> (w284:T2)
            n225 = Increment(x=w320) -> (x+1=w319:i32)
            n226 = Array Subset "M"(array=w330, index=w319) -> (w282:dbl[])  [unwired: 1 in]
            n227 = Array Subset "n"(array=w331, index=w319) -> (w313:dbl[])  [unwired: 1 in]
            n228 = Array Max & Min "Mmax"(array=w282) -> (max value=w280:dbl, max index (indices)=w316:i32)  [unwired: 2 out]
            n229 = Array Max & Min "nmax [1/min]"(array=w313) -> (max value=w278:dbl)  [unwired: 3 out]
            n230 = Array Subset "P"(array=w329, index=w319) -> (w314:dbl[])  [unwired: 1 in]
            n231 = Index Array "n(Mmax)"(array=w313, index=w316) -> (element=w310:dbl)
            n232 = Array Max & Min "Pmax"(array=w314) -> (max value=w311:dbl, max index (indices)=w315:i32)  [unwired: 2 out]
            n233 = case shown="\"Vario (km/h)\"" w284 {
              tunnel: [w341 w343] -> w283
              tunnel: w282 -> [w341 _]
              tunnel: w281 -> [_ w343]
              tunnel: w280 -> [w340 _]
              tunnel: [w340 w342] -> w279
              tunnel: w277 -> [_ w342]
              frame Default {
              }
              frame "Vario (km/h)" {
              }
            }
            n234 = Index Array "n(Pmax)"(array=w313, index=w315) -> (element=w301:dbl)
            n235 = Divide(x=w278, y=w302) -> (x/y=w328:dbl)
            n236 = call "n2v (SubVI).vi"("Übersetzung ermitteln aus"=w284, "Array (Eingang)"=w313, "Rollenumfang [m]"=w295) -> ("Array (Ausgang)"=w312:dbl[], "Boolesch"=w297:bool)  [unwired: 7 in]
            n237 = local read "Lufttemperatur [°C]"() -> (w307:dbl)
            n238 = local read "Luftdruck [mbar]"() -> (w306:dbl)
            n239 = Format Into String(format string="%.1f PS" ("Format-String"), w311) -> (resulting string=→"Pmax":string)  [unwired: 2 in, 1 out]
            n240 = Compound Arithmetic op=MULTIPLY "v(Pmax)"(w301, w295, w296) -> (w303:dbl)
            n241 = Compound Arithmetic op=MULTIPLY "vmax"(w328, w295, w296) -> (w309:dbl)
            n242 = Format Date/Time String(time format string (%c)="%x %H:%M ") -> (date/time string=w305:string)  [unwired: 2 in]
            n243 = Format Into String(format string="%.1f PS bei %d 1/min   |   %.1f Nm bei %d 1/min   |   vmax: %d km/h\\nDIN 70020 k =%.3f (%d \\B0C, %d mbar)\\n%s" ("Format-String"), w311, w301, w280, w310, w309, w308, w307, w306, w305) -> (resulting string=w300:string)  [unwired: 2 in, 1 out]
            n244 = Format Into String(format string="%.1f PS bei %d km/h   |   vmax: %d km/h\\nDIN 70020 k =%.3f (%d \\B0C, %d mbar)\\n%s" ("Format-String"), w311, w303, w309, w308, w307, w306, w305) -> (resulting string=w298:string)  [unwired: 2 in, 1 out]
            n245 = Bundle("Array (Ausgang)"=w312, w314) -> (w318:cluster{"Array (Ausgang)":dbl[], dbl[]})  [unwired: 1 in]
            n246 = Bundle("Array (Ausgang)"=w312, w283) -> (w317:cluster{"Array (Ausgang)":dbl[], dbl[]})  [unwired: 1 in]
            n247 = control-ref of="XY-Graph"() -> (w294:refnum<vi>)
            n248 = Multiply(x=1.8, y=w279) -> (x*y=w292:dbl)
            n249 = Select(t=w298, s=w297, f=w300) -> (s? t:f=→"Ergebnis":string)
            n250 = Build Array(w318, w317) -> (→"XY-Graph":cluster{"Array (Ausgang)":dbl[], dbl[]}[])
            n251 = property on="Eigenschaftsknoten" class="XYGraph (strikt)"(reference=w294, "ActYScl"=w286, "YScale.ScaleFit"=w293, "XScale.ScaleFit"=w293, "ActYScl"=w293, "YScale.Maximum"=w292, "YScale.Minimum"=w286) -> (reference out=w290:refnum<vi>)  [unwired: 1 in, 1 out]
            n252 = property on="Eigenschaftsknoten" class="XYGraph (strikt)"(reference=w290, "ActYScl"=w286) -> (reference out=w287:refnum<vi>, "YScale.Maximum"=w289:dbl)  [unwired: 1 in, 1 out]
            n253 = Add(x=w289, y=3.0) -> (x+y=w285:dbl)
            n254 = property on="Eigenschaftsknoten" class="XYGraph (strikt)"(reference=w287, "ActYScl"=w286, "YScale.Maximum"=w285) -> ()  [unwired: 1 in, 2 out]
            n255 = property on="Pmax" class="Str"("Text.FontSize"=48) -> ()  [unwired: 2 in, 2 out]
          }
        }
        n256 = flat-sequence {
          tunnel: w38 -> [w229]
          tunnel: w40 -> [w230]
          tunnel: w43 -> [w231]
          tunnel: w44 -> [w232]
          tunnel: w45 -> [w233]
          tunnel: w46 -> [w234]
          tunnel: w47 -> [w235]
          tunnel: w48 -> [w236]
          tunnel: [w236] -> w109
          tunnel: [w235] -> w108
          tunnel: [w234] -> w107
          tunnel: [w233] -> w106
          tunnel: [w232] -> w105
          tunnel: [w231] -> w104
          tunnel: [w230] -> w103
          tunnel: [w229] -> w102
          tunnel: [w225] -> w26
          tunnel: w25 -> [w225]
          tunnel: [w224] -> w17
          tunnel: w16 -> [w224]
          tunnel: w109 -> [w266]
          tunnel: w108 -> [w265]
          tunnel: w107 -> [w264]
          tunnel: w106 -> [w263]
          tunnel: w105 -> [w262]
          tunnel: w104 -> [w261]
          tunnel: w103 -> [w260]
          tunnel: w102 -> [w259]
          tunnel: w26 -> [w243]
          tunnel: w17 -> [w237]
          frame #0 {
            w227 = FALSE ("Start [F1]")
            w228 = 0  # Aktivieren
            n257 = local write "Start"(w227) -> ()
            n258 = property on="Drucken" class="Bool. (strikt)"("DisabledEnum"=w228) -> ()  [unwired: 2 in, 2 out]
            n259 = property on="Übersetzung ermitteln aus" class="Enum (strikt)"("DisabledEnum"=w228) -> ()  [unwired: 2 in, 2 out]
            n260 = property on="Speichern" class="Bool. (strikt)"("DisabledEnum"=w228) -> ()  [unwired: 2 in, 2 out]
            n261 = property on="Konfiguration:" class="Bool. (strikt)"("DisabledEnum"=w228) -> ()  [unwired: 2 in, 2 out]
            n262 = property on="Ende" class="Bool. (strikt)"("DisabledEnum"=w228) -> ()  [unwired: 2 in, 2 out]
            n263 = property on="Untersetzung\nermittelt" class="Bool. (strikt)"("BoolText.Text"="GO" ("Boolescher Text.Text"), "Blinking"=w227) -> ()  [unwired: 2 in, 2 out]
            n264 = local write "Untersetzung\nermittelt"(w227) -> ()
          }
          frame #1 {
            w238 = dbl[] []
            w241 = 0.0
            n265 = disable-structure shown="Deaktiviert" {
              frame Disabled {
                n266 = property on="XY-Graph" class="XYGraph (strikt)"("ActYScl"=0, "ActYScl"=1) -> ("XScale.Maximum"=w272:dbl, "XScale.Minimum"=w271:dbl, "YScale.Maximum"=w270:dbl, "YScale.Minimum"=w269:dbl, "YScale.Maximum"=w268:dbl, "YScale.Minimum"=w267:dbl)  [unwired: 2 in, 2 out]
                n267 = Build Array(w272, w271, w270, w269, w268, w267) -> ()  [unwired: 1 out]
              }
              frame Enabled {
              }
            }
            n268 = local read "Gleitender Mittelwert"() -> (w252:u8)
            n269 = local read "Differenzenquotient"() -> (w251:u8)
            n270 = local read "Übersetzung ermitteln aus"() -> (w248:T2)
            n271 = local read "Rollenträgheit [kgm²]"() -> (w256:dbl)
            n272 = local read "Messung Klimadaten"() -> (w245:bool)
            n273 = local read "Rollengeber [Inkr/U]"() -> (w257:u16)
            n274 = local read "Lufttemperatur [°C]"() -> (w250:dbl)
            n275 = local read "Reifenumfang [m]"() -> (w253:dbl)
            n276 = local read "n vom Gas [1/min]"() -> (w246:dbl)
            n277 = local read "Zündung [Imp/U]"() -> (w255:dbl)
            n278 = local read "v vom Gas [km/h]"() -> (w240:dbl)
            n279 = local read "Luftdruck [mbar]"() -> (w249:dbl)
            n280 = local read "nKuWe/nRolle"() -> (w242:dbl)
            n281 = local read "Getriebe [1:]"() -> (w254:dbl)
            n282 = local read "Dauer [s]"() -> (w247:dbl)
            n283 = Bundle("Fahrzeugdaten"="Fahrzeugdaten", "date/time string"=w263, "Rollengeber [Inkr/U]"=w257, "Rollenumfang [m]"=w261, "Rollenträgheit [kgm²]"=w256, "Zündung [Imp/U]"=w255, "Getriebe [1:]"=w254, "Reifenumfang [m]"=w253, "mean value"=w264, "Gleitender Mittelwert"=w252, "Differenzenquotient"=w251, u8 0, w266, "Numerisch"=w262, "Lufttemperatur [°C]"=w250, w241, "Luftdruck [mbar]"=w249, w265, w237, w238, w238, "Übersetzung ermitteln aus"=w248, "Dauer [s]"=w247, w241, w241, "n vom Gas [1/min]"=w246, w260, w259, "Messung Klimadaten"=w245, "VISA-Referenz (Ausgang)"=w243, "nKuWe/nRolle"=w242, "v vom Gas [km/h]"=w240) -> (→"Datenspeicher":T5)  [unwired: 1 in]
          }
        }
      }
    }
    n284 = Boolean To (0,1)(Boolean=w10) -> (0, 1=w12:i16)
    n285 = property on="Registerkarte 2" class="RKElem (strikt)"("Value"=w12) -> ()  [unwired: 2 in, 2 out]
    n286 = local read "Ende"() -> (w13:bool)
  }
  n287 = flat-sequence {
    frame #0 {
      n288 = local read "Datenspeicher"() -> (w727:T3)
      n289 = call <vilib>:"Application Directory.vi"() -> ("Application Directory"=w750:path)
      n290 = Build Path(base path=w750, name or relative path="Konfig.xml") -> (appended path=w729:path)
      n291 = call "LoadCluster(SubVI)2.0.5.vi"("Datenspeicher"=w727, "XML File Path"=w729) -> ("Value"=w728:T3)  [unwired: 8 in, 1 out]
      n292 = property on="Datenspeicher" class="Cluster (strikt)"("Value"=w728) -> ()  [unwired: 2 in, 2 out]
      n293 = Unbundle(w728) -> ("Fahrzeugdaten"=w748:string, "Rolle [Inkr/U]"=w747:u16, "Rollenumfang [m]"=w746:dbl, "Rollenträgheit [kgm²]"=w745:dbl, "Zündung [Imp/U]"=w744:dbl, "Getriebe [1:]"=w743:dbl, "Reifenumfang [m]"=w742:dbl, "element"=w733:dbl, "Gl. Mittelwert"=w741:u8, "Differenzenquotient"=w740:u8, "Lufttemperatur [°C]"=w739:dbl, "Luftdruck [mbar]"=w738:dbl, "Übersetzung ermitteln aus"=w735:u8, "[s]"=w737:dbl, "n vom Gas [1/min]"=w736:dbl, "Boolesch"=w734:bool, "Serielle Schnittstelle"=w732:refnum<visa-resource-name>, "nKuWe/nRolle"=w731:dbl, "v vom Gas [km/h]"=w730:dbl)  [unwired: 13 out]
      n294 = property on="Dauer [s]" class="DigWert (strikt)"("Value"=w737) -> ()  [unwired: 2 in, 2 out]
      n295 = property on="Fahrzeugdaten" class="Str"("Value"=w748) -> ()  [unwired: 2 in, 2 out]
      n296 = property on="Rollengeber [Inkr/U]" class="DigWert (strikt)"("Value"=w747) -> ()  [unwired: 2 in, 2 out]
      n297 = property on="Rollenumfang [m]" class="DigWert (strikt)"("Value"=w746) -> ()  [unwired: 2 in, 2 out]
      n298 = property on="Rollenträgheit [kgm²]" class="DigWert (strikt)"("Value"=w745) -> ()  [unwired: 2 in, 2 out]
      n299 = property on="Zündung [Imp/U]" class="DigWert (strikt)"("Value"=w744) -> ()  [unwired: 2 in, 2 out]
      n300 = property on="Getriebe [1:]" class="DigWert (strikt)"("Value"=w743) -> ()  [unwired: 2 in, 2 out]
      n301 = property on="Reifenumfang [m]" class="DigWert (strikt)"("Value"=w742) -> ()  [unwired: 2 in, 2 out]
      n302 = property on="nKuWe/nRolle" class="DigWert (strikt)"("Value"=w733) -> ()  [unwired: 2 in, 2 out]
      n303 = property on="Gleitender Mittelwert" class="DigWert (strikt)"("Value"=w741) -> ()  [unwired: 2 in, 2 out]
      n304 = property on="Differenzenquotient" class="DigWert (strikt)"("Value"=w740) -> ()  [unwired: 2 in, 2 out]
      n305 = property on="Lufttemperatur [°C]" class="DigWert (strikt)"("Value"=w739) -> ()  [unwired: 2 in, 2 out]
      n306 = property on="Luftdruck [mbar]" class="DigWert (strikt)"("Value"=w738) -> ()  [unwired: 2 in, 2 out]
      n307 = property on="Übersetzung ermitteln aus" class="Enum (strikt)"("Val(Sgnl)"=w735) -> ()  [unwired: 2 in, 2 out]
      n308 = property on="n vom Gas [1/min]" class="DigWert (strikt)"("Value"=w736) -> ()  [unwired: 2 in, 2 out]
      n309 = property on="Messung Klimadaten" class="Bool. (strikt)"("Val(Sgnl)"=w734) -> ()  [unwired: 2 in, 2 out]
      n310 = local write "Serielle Schnittstelle"(w732) -> ()
      n311 = property on="nKuWe/nRolle" class="DigWert (strikt)"("Value"=w731) -> ()  [unwired: 2 in, 2 out]
      n312 = property on="v vom Gas [km/h]" class="DigWert (strikt)"("Value"=w730) -> ()  [unwired: 2 in, 2 out]
      n313 = disable-structure shown="Deaktiviert" {
        disable-tunnel: _ -> [w754 _]
        frame Disabled {
          n314 = Array Size(array=w754) -> (size(s)=w753:i32)
          n315 = Equal?(x=w753, y=6) -> (x = y?=w752:bool)
          n316 = case shown="True" w752 {
            tunnel: w754 -> [_ w755]
            frame False {
            }
            frame True {
              n317 = Index Array(array=w755, index=2) -> (element=w759)
              n318 = Index Array(array=w755, index=0) -> (element=w762)
              n319 = Index Array(array=w755, index=4) -> (element=w756)
              n320 = Greater Than 0?(x=w759) -> (x > 0?=w760:bool)
              n321 = Greater Than 0?(x=w762) -> (x > 0?=w763:bool)
              n322 = Greater Than 0?(x=w756) -> (x > 0?=w757:bool)
              n323 = case shown="True" w760 {
                tunnel: w759 -> [_ w771]
                tunnel: w755 -> [_ w773]
                frame False {
                }
                frame True {
                  n324 = Index Array(array=w773, index=3) -> (element=w770)
                  n325 = property on="XY-Graph" class="XYGraph (strikt)"("ActYScl"=0, "YScale.Maximum"=w771, "YScale.Minimum"=w770) -> ()  [unwired: 2 in, 2 out]
                }
              }
              n326 = case shown="True" w763 {
                tunnel: w762 -> [_ w778]
                tunnel: w755 -> [_ w776]
                frame False {
                }
                frame True {
                  n327 = Index Array(array=w776, index=1) -> (element=w775)
                  n328 = property on="XY-Graph" class="XYGraph (strikt)"("XScale.Maximum"=w778, "XScale.Minimum"=w775) -> ()  [unwired: 2 in, 2 out]
                }
              }
              n329 = case shown="True" w757 {
                tunnel: w756 -> [_ w766]
                tunnel: w755 -> [_ w768]
                frame False {
                }
                frame True {
                  n330 = Index Array(array=w768, index=5) -> (element=w765)
                  n331 = property on="XY-Graph" class="XYGraph (strikt)"("ActYScl"=1, "YScale.Maximum"=w766, "YScale.Minimum"=w765) -> ()  [unwired: 2 in, 2 out]
                }
              }
            }
          }
        }
        frame Enabled {
        }
      }
    }
    frame #1 {
      w785 = 2  # Deaktivieren
      w787 = 0.0  # Graphen löschen
      n332 = local read "Serielle Schnittstelle"() -> (w783:refnum<visa-resource-name>)
      n333 = property on="Füllstand Lesepuffer" class="Schieber (strikt)"("Scale.Maximum"=100) -> ()  [unwired: 2 in, 2 out]
      n334 = property on="Frontpanel-Position" class="Bereich"("Origin"=T6 {"Horizontal"=8, "Vertical"=6}) -> ()  [unwired: 2 in, 2 out]
      n335 = property on="Drucken" class="Bool. (strikt)"("DisabledEnum"=w785) -> ()  [unwired: 2 in, 2 out]
      n336 = property on="Speichern" class="Bool. (strikt)"("DisabledEnum"=w785) -> ()  [unwired: 2 in, 2 out]
      n337 = Build Array(w787) -> (w786:dbl[])
      n338 = VISA Clear(VISA resource name=w783) -> (VISA resource name out=w782:refnum<visa-resource-name>, error out=w781:errorcluster)  [unwired: 1 in]
      n339 = property on="Untersetzung-Graph" class="SVDiagr (strikt)"("History Data"=w786) -> ()  [unwired: 2 in, 2 out]
      n340 = VISA Close(VISA resource name=w782, error in (no error)=w781) -> (error out=w780:errorcluster)
      n341 = case shown="Kein Fehler" w780 {
        tunnel: [T4."Enabled" ("Deaktiviert") T4."Disabled and Grayed Out" ("Deaktiviert")] -> w779
        frame No Error {
        }
        frame Error {
        }
      }
      n342 = property on="Start" class="Bool. (strikt)"("DisabledEnum"=w779) -> ()  [unwired: 2 in, 2 out]
    }
  }
  n343 = while {
    stop <- w794 stop-if-true
    n344 = event shown="[8] \"Übersetzung ermitteln aus\": Wertänderung" {
      selector: _ -> [_ _ _ _ _ _ _ _ _ _]
      dyn-events: _ -> [_ _ _ _ _ _ _ _ _ _]
      timeout: _ -> [_ _ _ _ _ _ _ _ _ _]
      tunnel: [_ _ _ TRUE _ _ _ _ _ _] -> w794
      event "Konfiguration:": Value Change {
        n345 = event-data() -> ("OldVal"=w796:bool)  [unwired: 1 in, 5 out]
        n346 = flat-sequence {
          tunnel: [w817] -> w797
          tunnel: w796 -> [w817]
          tunnel: w797 -> [w818]
          frame #0 {
            n347 = property on="Datenspeicher" class="Cluster (strikt)"() -> ("Value"=w816:T3)  [unwired: 2 in, 2 out]
            n348 = call "LoadCluster(SubVI)2.0.5.vi"("Datenspeicher"=w816) -> ("Value"=w815:T3)  [unwired: 9 in, 1 out]
            n349 = Unbundle(w815) -> ("Fahrzeugdaten"=w814:string, "Rolle [Inkr/U]"=w813:u16, "Rollenumfang [m]"=w812:dbl, "Rollenträgheit [kgm²]"=w811:dbl, "Zündung [Imp/U]"=w810:dbl, "Getriebe [1:]"=w809:dbl, "Reifenumfang [m]"=w808:dbl, "Gl. Mittelwert"=w807:u8, "Differenzenquotient"=w806:u8, "Lufttemperatur [°C]"=w805:dbl, "Luftdruck [mbar]"=w804:dbl, "Übersetzung ermitteln aus"=w801:u8, "[s]"=w803:dbl, "n vom Gas [1/min]"=w802:dbl, "Boolesch"=w800:bool, "nKuWe/nRolle"=w799:dbl, "v vom Gas [km/h]"=w798:dbl)  [unwired: 15 out]
            n350 = property on="Dauer [s]" class="DigWert (strikt)"("Value"=w803) -> ()  [unwired: 2 in, 2 out]
            n351 = property on="Fahrzeugdaten" class="Str"("Value"=w814) -> ()  [unwired: 2 in, 2 out]
            n352 = property on="Rollengeber [Inkr/U]" class="DigWert (strikt)"("Value"=w813) -> ()  [unwired: 2 in, 2 out]
            n353 = property on="Rollenumfang [m]" class="DigWert (strikt)"("Value"=w812) -> ()  [unwired: 2 in, 2 out]
            n354 = property on="Rollenträgheit [kgm²]" class="DigWert (strikt)"("Value"=w811) -> ()  [unwired: 2 in, 2 out]
            n355 = property on="Zündung [Imp/U]" class="DigWert (strikt)"("Value"=w810) -> ()  [unwired: 2 in, 2 out]
            n356 = property on="Getriebe [1:]" class="DigWert (strikt)"("Value"=w809) -> ()  [unwired: 2 in, 2 out]
            n357 = property on="Reifenumfang [m]" class="DigWert (strikt)"("Value"=w808) -> ()  [unwired: 2 in, 2 out]
            n358 = property on="Gleitender Mittelwert" class="DigWert (strikt)"("Value"=w807) -> ()  [unwired: 2 in, 2 out]
            n359 = property on="Lufttemperatur [°C]" class="DigWert (strikt)"("Value"=w805) -> ()  [unwired: 2 in, 2 out]
            n360 = property on="Luftdruck [mbar]" class="DigWert (strikt)"("Value"=w804) -> ()  [unwired: 2 in, 2 out]
            n361 = property on="n vom Gas [1/min]" class="DigWert (strikt)"("Value"=w802) -> ()  [unwired: 2 in, 2 out]
            n362 = property on="Messung Klimadaten" class="Bool. (strikt)"("Val(Sgnl)"=w800) -> ()  [unwired: 2 in, 2 out]
            n363 = property on="nKuWe/nRolle" class="DigWert (strikt)"("Value"=w799) -> ()  [unwired: 2 in, 2 out]
            n364 = property on="v vom Gas [km/h]" class="DigWert (strikt)"("Value"=w798) -> ()  [unwired: 2 in, 2 out]
            n365 = property on="Differenzenquotient" class="DigWert (strikt)"("Value"=w806) -> ()  [unwired: 2 in, 2 out]
            n366 = property on="Übersetzung ermitteln aus" class="Enum (strikt)"("Val(Sgnl)"=w801) -> ()  [unwired: 2 in, 2 out]
          }
          frame #1 {
            n367 = property on="Konfiguration:" class="Bool. (strikt)"("Value"=w818) -> ()  [unwired: 2 in, 2 out]
          }
        }
      }
      event "Drucken": Value Change {
        n368 = event-data() -> ("OldVal"=w819:bool)  [unwired: 1 in, 5 out]
        n369 = flat-sequence {
          tunnel: [w824] -> w820
          tunnel: w819 -> [w824]
          tunnel: w820 -> [w825]
          frame #0 {
            n370 = control-ref of="Fahrzeugdaten"() -> (w822:refnum<vi>)
            n371 = control-ref of="XY-Graph"() -> (w823:refnum<vi>)
            n372 = control-ref of="Ergebnis"() -> (w821:refnum<vi>)
            n373 = call "printgraph_V0.01.vi"("reference 2"=w821, "Fahrzeugdaten"=w822, "XYGraph (Eingang)"=w823) -> ()  [unwired: 9 in]
          }
          frame #1 {
            n374 = property on="Drucken" class="Bool. (strikt)"("Value"=w825) -> ()  [unwired: 2 in, 2 out]
          }
        }
      }
      event "Speichern": Value Change {
        n375 = event-data() -> ("OldVal"=w827:bool)  [unwired: 1 in, 5 out]
        n376 = control-ref of="Datenspeicher"() -> (w826:refnum<vi>)
        n377 = local write "Speichern"(w827) -> ()
        n378 = call "savecluster_V0.01.vi"("Datenspeicher 2"=w826) -> ()  [unwired: 2 in]
      }
      event "Ende": Value Change {
        w835 = 0.0 ("element")
        n379 = event-data() -> ("OldVal"=w833:bool)  [unwired: 1 in, 5 out]
        n380 = local read "Datenspeicher"() -> (w836:T3)
        n381 = flat-sequence {
          tunnel: w833 -> [w867]
          tunnel: [w867] -> w832
          frame #0 {
            n382 = Wait (ms)(milliseconds to wait=u32 200) -> ()  [unwired: 1 out]
          }
        }
        n383 = Unbundle By Name(w836) -> ("Rolle [Inkr/U]"=w857:u16, "Rollenumfang [m]"=w856:dbl, "Rollenträgheit [kgm²]"=w855:dbl, "Zündung [Imp/U]"=w854:dbl, "Getriebe [1:]"=w853:dbl, "Reifenumfang [m]"=w852:dbl, "Gl. Mittelwert"=w851:u8, "Differenzenquotient"=w850:u8, "Fahrzeugdaten"=w849:string, "Lufttemperatur [°C]"=w848:dbl, "Luftfeuchtigkeit [%]"=w847:dbl, "Luftdruck [mbar]"=w845:dbl, "nRolle"=w846:dbl[], "Übersetzung ermitteln aus"=w844:u8, "[s]"=w843:dbl, "nmin [1/min]"=w842:dbl, "nmax [1/min]"=w841:dbl, "n vom Gas [1/min]"=w840:dbl, "Boolesch"=w839:bool, "Serielle Schnittstelle"=w834:refnum<visa-resource-name>, "nWelle"=w831:dbl[], "ArrayReserve1"=w829:dbl[], "ArrayReserve2"=w828:dbl[], "v vom Gas [km/h]"=w830:dbl)  [unwired: 3 out]
        n384 = call <vilib>:"Application Directory.vi"() -> ("Application Directory"=w862:path)
        n385 = local write "Ende"(w832) -> ()
        n386 = Bundle By Name(cluster=w836, "Fahrzeugdaten"="", "date/time string"="", "Rolle [Inkr/U]"=w857, "Rollenumfang [m]"=w856, "Rollenträgheit [kgm²]"=w855, "Zündung [Imp/U]"=w854, "Getriebe [1:]"=w853, "Reifenumfang [m]"=w852, "element"=0.0, "Gl. Mittelwert"=w851, "Differenzenquotient"=w850, "Fahrzeugdaten"=w849, "element"=w835, "element"=w835, "Lufttemperatur [°C]"=w848, "Luftfeuchtigkeit [%]"=w847, "Luftdruck [mbar]"=w845, "nRolle"=w846, "Übersetzung ermitteln aus"=w844, "[s]"=w843, "nmin [1/min]"=w842, "nmax [1/min]"=w841, "n vom Gas [1/min]"=w840, "Boolesch"=w839, "Serielle Schnittstelle"=w834, "nWelle"=w831, "ArrayReserve1"=w829, "ArrayReserve2"=w828, "v vom Gas [km/h]"=w830) -> (w837:T3)
        n387 = Build Path(base path=w862, name or relative path="Konfig.xml") -> (appended path=w860:path)
        n388 = Flatten To XML(anything=w837) -> (xml string=w864:string)
        n389 = call-poly <vilib>:"Write to XML File.vi"("XML Input"=w864, "XML File Path"=w860) -> ("error out"=w863:errorcluster)  [unwired: 7 in, 2 out]
        n390 = case shown="Kein Fehler" w863 {
          frame No Error {
          }
          frame Error {
          }
        }
      }
      event "Serielle Schnittstelle": Value Change {
        n391 = event-data() -> ()  [unwired: 1 in, 6 out]
        n392 = property on="Start" class="Bool. (strikt)"("DisabledEnum"=T4."Enabled" ("Deaktiviert")) -> ()  [unwired: 2 in, 2 out]
      }
      event "Messung Klimadaten": Value Change {
        n393 = event-data() -> ("NewVal"=w869:bool)  [unwired: 1 in, 5 out]
        n394 = case shown="True" w869 {
          frame True {
            w870 = T4."Disabled and Grayed Out" ("Deaktiviert")
            n395 = property on="Lufttemperatur [°C]" class="DigWert (strikt)"("DisabledEnum"=w870) -> ()  [unwired: 2 in, 2 out]
            n396 = property on="Luftdruck [mbar]" class="DigWert (strikt)"("DisabledEnum"=w870) -> ()  [unwired: 2 in, 2 out]
          }
          frame False {
            w871 = T4."Enabled" ("Deaktiviert")
            n397 = property on="Lufttemperatur [°C]" class="DigWert (strikt)"("DisabledEnum"=w871) -> ()  [unwired: 2 in, 2 out]
            n398 = property on="Luftdruck [mbar]" class="DigWert (strikt)"("DisabledEnum"=w871) -> ()  [unwired: 2 in, 2 out]
          }
        }
      }
      event "Spenden": Value Change {
        n399 = event-data() -> ()  [unwired: 1 in, 6 out]
        n400 = case shown="True" "Spenden" {
          frame False {
          }
          frame True {
            n401 = call-poly <vilib>:"Open URL in Default Browser.vi"("URL"="https://www.paypal.com/cgi-bin/webscr?cmd=_s-xclick&hosted_button_id=8SA7Y5J5P5N3W&source=url") -> ()  [unwired: 5 in, 2 out]
          }
        }
      }
      event "Recalc": Value Change {
        n402 = event-data() -> ("OldVal"=w876:bool)  [unwired: 1 in, 5 out]
        n403 = property on="Recalc" class="Bool. (strikt)"("Value"=w876) -> ()  [unwired: 2 in, 2 out]
        n404 = property on="Datenspeicher" class="Cluster (strikt)"() -> ("Value"=w874:T3)  [unwired: 2 in, 2 out]
        n405 = call "ReCalc_V2.00.vi"("Berechnen"=TRUE, "Datenspeicher"=w874) -> ()  [unwired: 3 in]
      }
      event "Übersetzung ermitteln aus": Value Change {
        n406 = event-data() -> ("NewVal"=w891:T2)  [unwired: 1 in, 5 out]
        n407 = case shown="\"Vario (km/h)\"" w891 {
          tunnel: [w908 w909 w911 w914] -> w892
          tunnel: [w908 w910 w911 w913] -> w887
          tunnel: [w908 w909 w912 w913] -> w886
          tunnel: [w908 w910 w912 w914] -> w885
          tunnel: [T4."Enabled" ("Deaktiviert") w909 w911 w913] -> w884
          frame "Vario (km/h)" {
            w908 = T4."Disabled and Grayed Out" ("Deaktiviert")
          }
          frame "nKuWe / nRolle" {
            w910 = T4."Enabled" ("Deaktiviert")
            w909 = T4."Disabled and Grayed Out" ("Deaktiviert")
          }
          frame "Zündsignal", Default {
            w912 = T4."Enabled" ("Deaktiviert")
            w911 = T4."Disabled and Grayed Out" ("Deaktiviert")
          }
          frame "Getriebe & Reifen" {
            w913 = T4."Disabled and Grayed Out" ("Deaktiviert")
            w914 = T4."Enabled" ("Deaktiviert")
          }
        }
        n408 = case shown="\"Vario (km/h)\"" w891 {
          tunnel: [TRUE w901] -> w880
          tunnel: ["n [1/min]" "M [Nm]"] -> w890
          tunnel: [200.0 14000.0] -> w889
          tunnel: ["v [km/h]" "n [1/min]"] -> w883
          tunnel: [14000.0 50.0] -> w882
          tunnel: [u32 16777216 w902] -> w879
          tunnel: [u32 16711680 w902] -> w878
          tunnel: [FALSE w901] -> w877
          frame "Vario (km/h)" {
          }
          frame Default {
            w902 = u32 9868950
            w901 = TRUE
          }
        }
        n409 = property on="XY-Graph" class="XYGraph (strikt)"("ActYScl"=1, "YScale.NameLbl.Text"=w890, "YScale.Maximum"=w882, "XScale.NameLbl.Text"=w883, "XScale.Maximum"=w889) -> ()  [unwired: 2 in, 2 out]
        n410 = property on="Text Zündung" class="Str"("Text.TextColor"=w878) -> ()  [unwired: 2 in, 2 out]
        n411 = property on="Welle [1/min]" class="Drehknopf (strikt)"("Visible"=w880, "Active Slider"=1, "FG Color"=w879) -> ()  [unwired: 2 in, 2 out]
        n412 = property on="Text Rolle" class="Str"("Visible"=w877) -> ()  [unwired: 2 in, 2 out]
        n413 = property on="nKuWe/nRolle" class="DigWert (strikt)"("DisabledEnum"=w887) -> ()  [unwired: 2 in, 2 out]
        n414 = property on="v vom Gas [km/h]" class="DigWert (strikt)"("DisabledEnum"=w884) -> ()  [unwired: 2 in, 2 out]
        n415 = property on="n vom Gas [1/min]" class="DigWert (strikt)"("DisabledEnum"=w885) -> ()  [unwired: 2 in, 2 out]
        n416 = property on="Getriebe [1:]" class="DigWert (strikt)"("DisabledEnum"=w892) -> ()  [unwired: 2 in, 2 out]
        n417 = property on="Reifenumfang [m]" class="DigWert (strikt)"("DisabledEnum"=w892) -> ()  [unwired: 2 in, 2 out]
        n418 = property on="Zündung [Imp/U]" class="DigWert (strikt)"("DisabledEnum"=w886) -> ()  [unwired: 2 in, 2 out]
        n419 = property on="Dauer [s]" class="DigWert (strikt)"("DisabledEnum"=w886) -> ()  [unwired: 2 in, 2 out]
      }
      event "Reset Skalierung": Value Change {
        w919 = 0.0
        n420 = event-data() -> ()  [unwired: 1 in, 6 out]
        n421 = local read "Übersetzung ermitteln aus"() -> (w917:T2)
        n422 = case shown="\"Vario (km/h)\"" w917 {
          tunnel: [14000.0 200.0] -> w916
          tunnel: [50.0 14000.0] -> w915
          frame Default {
          }
          frame "Vario (km/h)" {
          }
        }
        n423 = property on="XY-Graph" class="XYGraph (strikt)"("XScale.Maximum"=w916, "XScale.Minimum"=w919, "ActYScl"=w919, "YScale.Maximum"=30.0, "YScale.Minimum"=w919, "ActYScl"=1, "YScale.Maximum"=w915, "YScale.Minimum"=w919) -> ()  [unwired: 2 in, 2 out]
      }
    }
    n424 = property class="Anw"() -> ("App.Kind"=w792:T7)  [unwired: 2 in, 2 out]
    n425 = Greater?(x=w792, y=1) -> (0:w793:bool)
    n426 = case shown="True" w793 {
      tunnel: w794 -> [_ w795]
      frame False {
      }
      frame True {
        n427 = Quit LabVIEW(quit? (T)=w795) -> ()
      }
    }
  }
  "Text Zündung" <- "Zündung"
  "Text Rolle" <- "Rolle"
